vi "calc_noise_mask.vi"(4 "u8_ar_image_pixel_array":dbl[][][](array[numeric])) -> (1 "u8_ar_noise_mask":u8[][](array[numeric]), 2 "img_noise mask":T1(plugin-control))   [LabVIEW 2011]
uses:
  global_vars.vi
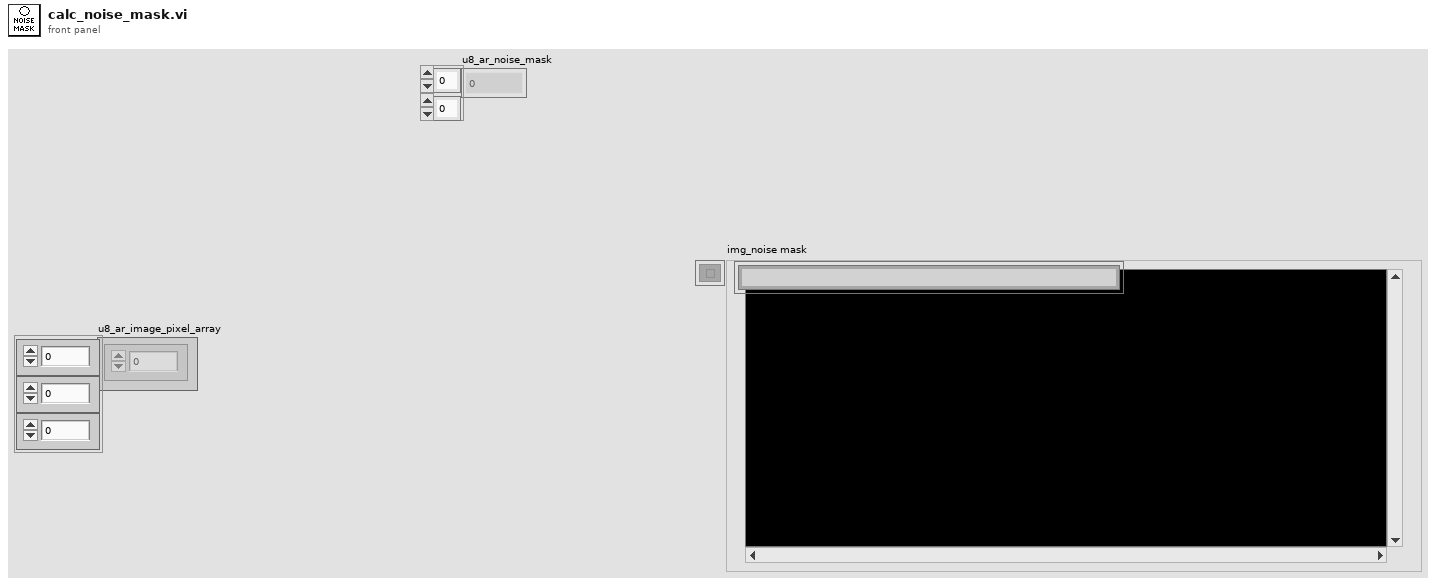
[diagram p1: front panel]
types:
  T1 = typedef "IMAQ Image.ctl" = refnum<image>
  T2 = typedef "Image Type" = u32
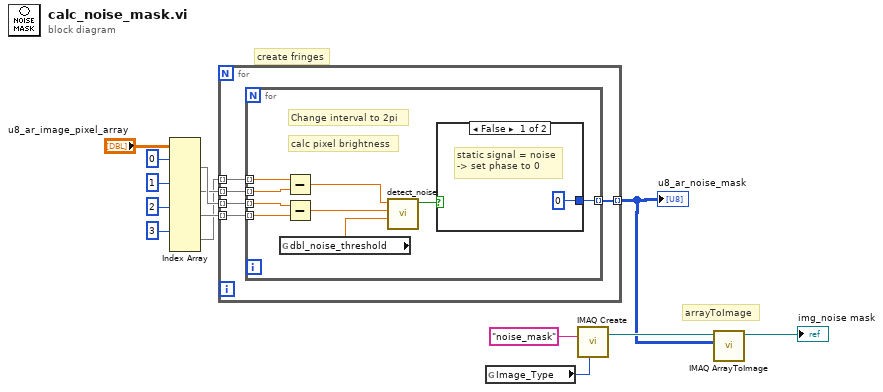
[diagram p0: block diagram]
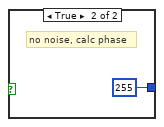
[diagram p2: hidden frame]
diagram:
  # "arrayToImage"
  # "create fringes"
  n1 = Index Array(array="u8_ar_image_pixel_array", index (dim 0) #1=0 ("index (page)"), index (dim 0) #2=1 ("index (page)"), index (dim 0) #3=2 ("index (page)"), index (dim 0) #4=3 ("index (page)")) -> (element #1=w10:dbl[][], element #2=w9:dbl[][], element #3=w8:dbl[][], element #4=w7:dbl[][])  [unwired: 8 in]
  n2 = for {
    tunnel: w10 -> [w19] mode=indexing
    tunnel: w9 -> [w18] mode=indexing
    tunnel: w8 -> [w17] mode=indexing
    tunnel: w7 -> [w16] mode=indexing
    tunnel: [w15] -> w1 mode=indexing
    n3 = for {
      tunnel: w19 -> [w28] mode=indexing
      tunnel: w18 -> [w27] mode=indexing
      tunnel: w17 -> [w26] mode=indexing
      tunnel: w16 -> [w25] mode=indexing
      tunnel: [w21] -> w15 mode=indexing
      # "Change interval to 2pi"
      # "calc pixel brightness"
      n4 = global read "global_vars.vi" "dbl_noise_threshold"() -> (w20:dbl)
      n5 = Subtract(x=w25, y=w27) -> (x-y=w23:dbl)
      n6 = Subtract(x=w28, y=w26) -> (x-y=w22:dbl)
      n7 = call "detect_noise.vi"("threshold"=w20, "i1-i3"=w22, "i4-i2"=w23) -> ("is signal"=w24:bool)  [unwired: 8 in]
      n8 = case shown="False" w24 {
        tunnel: [u8 0 u8 255] -> w21
        frame False {
          # "static signal = noise\n-> set phase to 0"
        }
        frame True {
          # "no noise, calc phase"
        }
      }
    }
  }
  "u8_ar_noise_mask" <- w1
  n9 = global read "global_vars.vi" "Image_Type"() -> (w2:T2)
  n10 = call "IMAQ Create"("Image Name"="noise_mask" ("image name"), "Image Type"=w2) -> ("New Image"=w3:T1)  [unwired: 2 in, 2 out]
  n11 = call "IMAQ ArrayToImage"("Image Pixels (U8)"=w1, "Image"=w3) -> ("Image Out"=→"img_noise mask":T1)  [unwired: 8 in, 1 out]
